vi "TIME UPDATE.vi"() -> ()   [LabVIEW 2017]
panel:
  out "AM/PM":string
  out "SEC":string
  out "MINUTE":string
  out "HOUR":string
  out "YEAR":string
  out "MONTH":string
  out "DATE":string
  in  "stop":bool
  out "time string":string
  out "date string":string
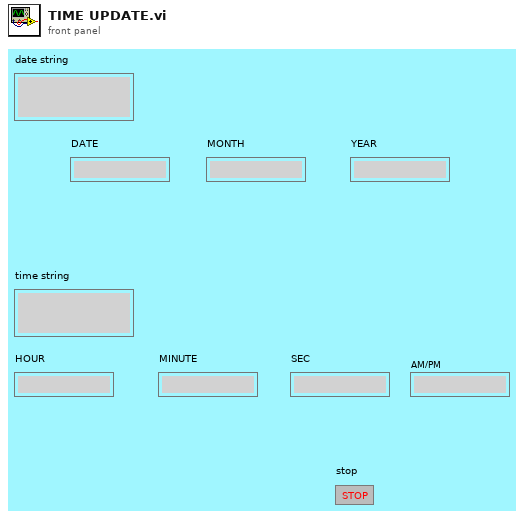
[diagram p1: front panel]
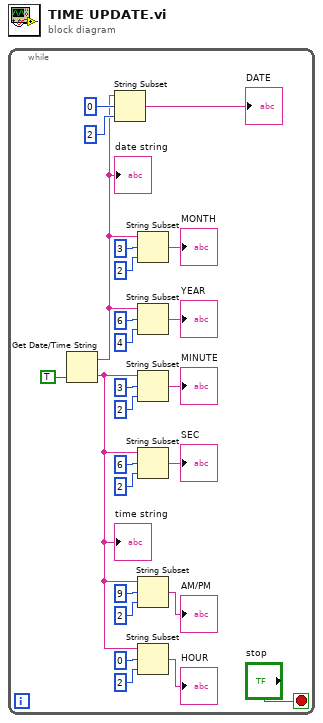
[diagram p0: block diagram]
diagram:
  n1 = while {
    stop <- "stop" stop-if-true
    n2 = Get Date/Time String(want seconds? (F)=TRUE) -> (date string=w8:string, time string=w2:string)  [unwired: 2 in]
    "date string" <- w8
    "time string" <- w2
    n3 = String Subset(string=w8, offset (0)=0, length (rest)=2 ("length (rest)")) -> (substring=→"DATE":string)
    n4 = String Subset(string=w8, offset (0)=3, length (rest)=2 ("length (rest)")) -> (substring=→"MONTH":string)
    n5 = String Subset(string=w8, offset (0)=6, length (rest)=4 ("length (rest)")) -> (substring=→"YEAR":string)
    n6 = String Subset(string=w2, offset (0)=3, length (rest)=2 ("length (rest)")) -> (substring=→"MINUTE":string)
    n7 = String Subset(string=w2, offset (0)=6, length (rest)=2 ("length (rest)")) -> (substring=→"SEC":string)
    n8 = String Subset(string=w2, offset (0)=9, length (rest)=2 ("length (rest)")) -> (substring=→"AM/PM":string)
    n9 = String Subset(string=w2, offset (0)=0, length (rest)=2 ("length (rest)")) -> (substring=→"HOUR":string)
  }
